vi "ChartRangeTest.vi"() -> ()   [LabVIEW 2018]
panel:
  out "Min Time String":timestamp format="%<%X\n%x>T"
  in  "Slide":cluster{dbl, dbl}(slide)={0.0, 5.05050505050505}
  out "Max Time String":timestamp format="%<%X\n%x>T"
  out "date/time string":string
  in  "View Subset":bool
  in  "stop":bool
  out "Waveform Chart":cluster{"Scalar":dbl, dbl, dbl, dbl}(graph)
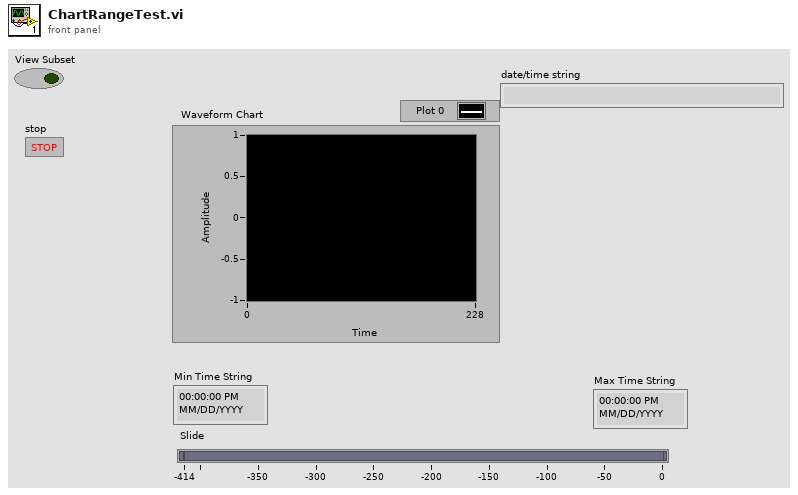
[diagram p1: front panel]
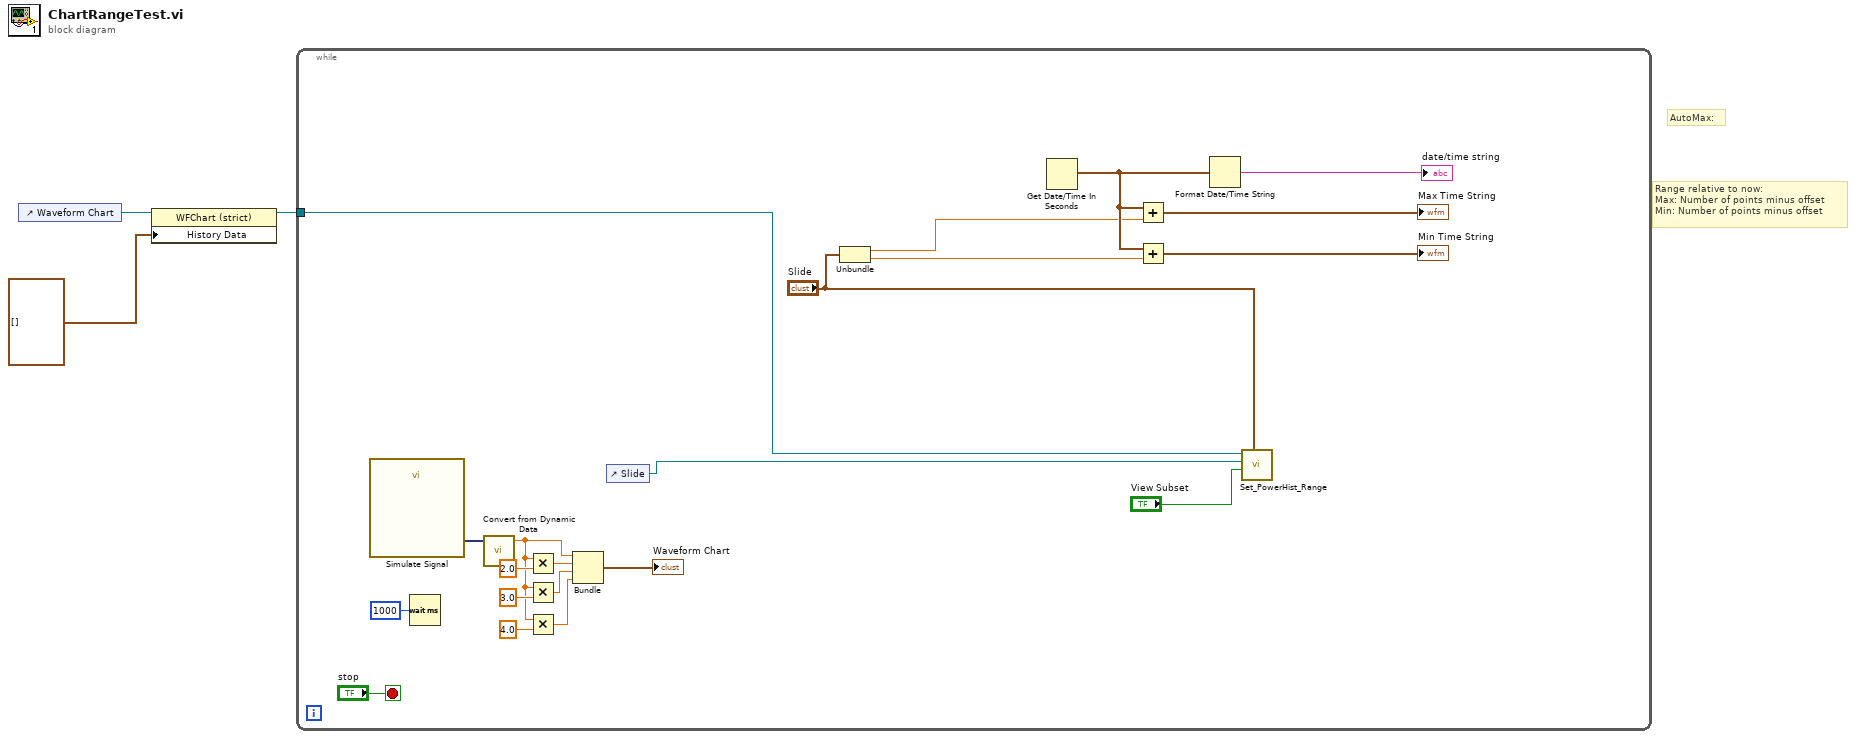
[diagram p0: block diagram]
diagram:
  # "Range relative to now: \nMax: Number of points minus offset\nMin: Number of points minus offset"
  # "AutoMax:"
  n1 = control-ref of="Waveform Chart"() -> (w3:refnum<vi>)
  n2 = property class="WFChart (strict)"(reference=w3, "History Data"=cluster{"Scalar":dbl, dbl, dbl, dbl}[] []) -> (reference out=w2:refnum<vi>)  [unwired: 1 in, 1 out]
  n3 = while {
    tunnel: w2 -> [w21]
    stop <- "stop" stop-if-true
    n4 = call "Simulate Signal"() -> ("Sine"=w24:dynamicdata)  [unwired: 14 in, 1 out]
    n5 = Wait (ms)(milliseconds to wait=u32 1000) -> ()  [unwired: 1 out]
    n6 = call "Convert from Dynamic Data"("Dynamic Data Type"=w24) -> ("Scalar"=w6:dbl)  [unwired: 3 in]
    n7 = Multiply(x=w6, y=2.0) -> (x*y=w8:dbl)
    n8 = Multiply(x=w6, y=3.0) -> (x*y=w7:dbl)
    n9 = Multiply(x=w6, y=4.0) -> (x*y=w5:dbl)
    n10 = Bundle("Scalar"=w6, w8, w7, w5) -> (→"Waveform Chart":cluster{"Scalar":dbl, dbl, dbl, dbl})  [unwired: 1 in]
    n11 = control-ref of="Slide"() -> (w15:refnum<vi>)
    n12 = Unbundle("Slide") -> (w14:dbl, w13:dbl)
    n13 = Get Date/Time In Seconds() -> (seconds since 1Jan1904=w16:timestamp)
    n14 = Add(x=w16, y=w14) -> (x+y=→"Max Time String":timestamp)
    n15 = Add(x=w16, y=w13) -> (x+y=→"Min Time String":timestamp)
    n16 = Format Date/Time String(seconds (now)=w16) -> (date/time string=→"date/time string":string)  [unwired: 2 in]
    n17 = call "Set_PowerHist_Range.vi"("Slide"="Slide", "View Subset"="View Subset", "Slide Ref"=w15, "ChartRef"=w21) -> ()  [unwired: 8 in]
  }
